vi "MathCAD wait until open.vi"(8 "error in (no error)":errorcluster) -> (0 "error out":errorcluster, 3 "Mathcad.IMathcadApplication":refnum<k7>)   [LabVIEW 2015, in "AguaClara Library.lvlib"]
uses:
  AguaClara Library.lvlib
panel:
  out "NaN/Path/Refnum? 2":bool
  out "NaN/Path/Refnum?":bool
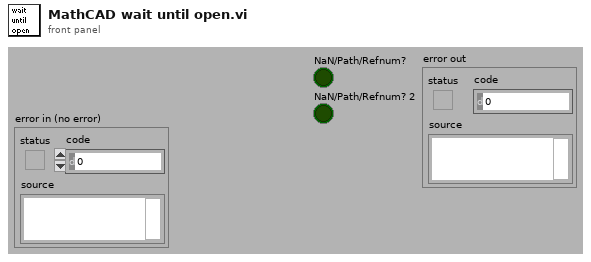
[diagram p1: front panel]
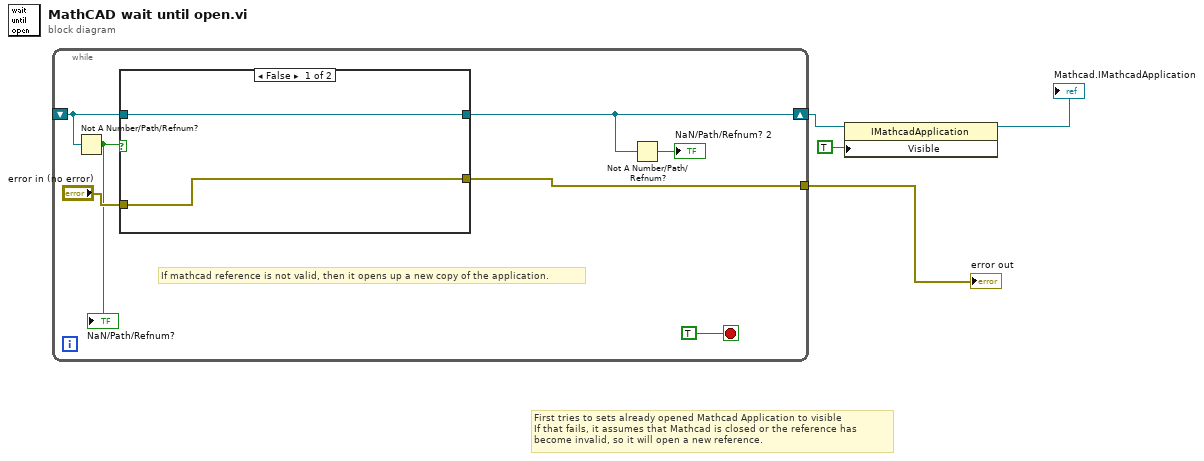
[diagram p0: block diagram]
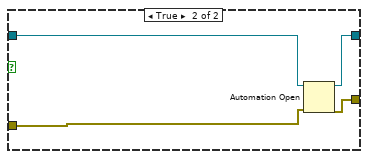
[diagram p2: hidden frame]
diagram:
  # "First tries to sets already opened Mathcad Application to visible\nIf that fails, it assumes that Mathcad is closed or the reference has become invalid, so it will open a new reference."
  n1 = while {
    shift-right: [w7] -> w3
    shift-left: _ -> [w9]
    tunnel: [w5] -> w4
    stop <- TRUE stop-if-true
    # "If mathcad reference is not valid, then it opens up a new copy of the application."
    n2 = Not A Number/Path/Refnum?(number/path/refnum=w9) -> (NaN/Path/Refnum?=w10:bool)
    "NaN/Path/Refnum?" <- w10
    n3 = case shown="False" w10 {
      tunnel: "error in (no error)" -> [w13 w14]
      tunnel: [w13 w16] -> w5
      tunnel: w9 -> [w12 w17]
      tunnel: [w12 w15] -> w7
      frame False {
      }
      frame True {
        n4 = Automation Open(error in (no error)=w14, Automation Refnum=w17) -> (Automation Refnum=w15:refnum<k7>, error out=w16:errorcluster)  [unwired: 2 in]
      }
    }
    n5 = Not A Number/Path/Refnum?(number/path/refnum=w7) -> (NaN/Path/Refnum?=→"NaN/Path/Refnum? 2":bool)
  }
  "error out" <- w4
  n6 = property class="IMathcadApplication"(reference=w3, "Visible"=TRUE) -> (reference out=→"Mathcad.IMathcadApplication":refnum<k7>)  [unwired: 1 in, 1 out]
